vi "GamepadTeleop.vi"   [LabVIEW 2014]
uses:
  Elevator System/Typedef/TeirNumber.ctl
  <vilib>/Rock Robotics/WPI/Joystick/WPI_JoystickGetSetRefNum.vi
  Elevator System/Elevator System.lvlib
types:
  T1 = typedef "WPI_JoystickDevRef.ctl" = cluster{"Device":T2}
  T2 = typedef "WPI_JoystickDeviceEnum.ctl" = enum16{"USB 0", "USB 1", "USB 2", "USB 3", "USB 4", "USB 5"}
  T3 = typedef "Elevator System.lvlib/TeirNumber.ctl" = enum16{"T1", "T2", "T3", "T4", "T5", "T6"}
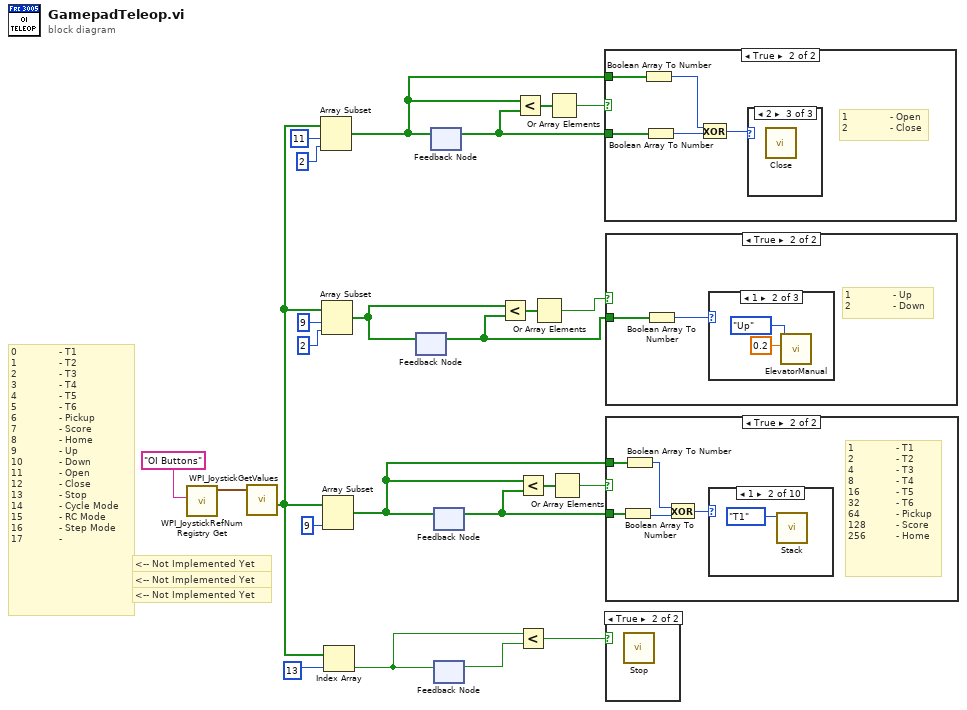
[diagram p0: block diagram]
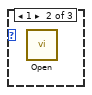
[diagram p4: hidden frame]
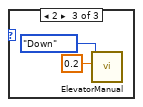
[diagram p8: hidden frame]
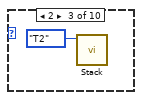
[diagram p11: hidden frame]
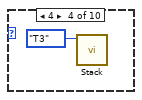
[diagram p12: hidden frame]
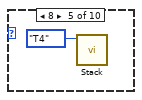
[diagram p13: hidden frame]
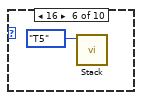
[diagram p14: hidden frame]
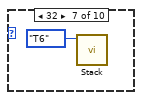
[diagram p15: hidden frame]
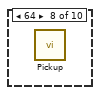
[diagram p16: hidden frame]
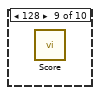
[diagram p17: hidden frame]
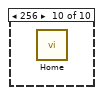
[diagram p18: hidden frame]
diagram:
  # "<-- Not Implemented Yet"
  # "<-- Not Implemented Yet"
  # "<-- Not Implemented Yet"
  # "0              - T1\n1              - T2\n2              - T3\n3              - T4\n4              - T5\n5              - T6\n6              - Pickup\n7              - Score\n8              - Home\n9              - Up\n10            - Down\n11            - Open\n12            - Close\n13            - Stop \n14            - Cycle Mode \n15            - RC Mode\n16            - Step Mode\n17            -"
  n1 = call <vilib>:"WPI_JoystickRefNum Registry Get.vi"("refnum name"="OI Buttons") -> ("JoystickDevRef"=w23:T1)  [unwired: 1 in, 9 out]
  n2 = call <vilib>:"WPI_JoystickGetValues.vi"("JoystickDevRef"=w23) -> ("Buttons"=w7:bool[])  [unwired: 6 in, 4 out]
  n3 = Array Subset(array=w7, index=11 ("length"), length=2) -> (w6:bool[])
  n4 = Array Subset(array=w7, index=9 ("length"), length=2) -> (w3:bool[])
  n5 = Array Subset(array=w7, length=9) -> (w5:bool[])  [unwired: 1 in]
  n6 = Index Array(array=w7, index=13) -> (element=w14:bool)
  n7 = feedback #1() -> (w1:bool[])  [unwired: 1 in]
  n8 = feedback-in #1(w3) -> ()
  n9 = feedback #2() -> (w9:bool[])  [unwired: 1 in]
  n10 = feedback-in #2(w6) -> ()
  n11 = feedback #3() -> (w20:bool[])  [unwired: 1 in]
  n12 = feedback-in #3(w5) -> ()
  n13 = feedback #4() -> (w15:bool)  [unwired: 1 in]
  n14 = feedback-in #4(w14) -> ()
  n15 = Less?(x=w3, y=w1) -> (x < y?=w4:bool[])
  n16 = Less?(x=w6, y=w9) -> (x < y?=w11:bool[])
  n17 = Less?(x=w5, y=w20) -> (x < y?=w22:bool[])
  n18 = Less?(x=w14, y=w15) -> (x < y?=w13:bool)
  n19 = Or Array Elements(Boolean array=w4) -> (logical OR=w2:bool)
  n20 = Or Array Elements(Boolean array=w11) -> (logical OR=w10:bool)
  n21 = Or Array Elements(Boolean array=w22) -> (logical OR=w21:bool)
  n22 = case shown="True" w10 {
    tunnel: w9 -> [_ w29]
    tunnel: w6 -> [_ w25]
    frame False {
    }
    frame True {
      # "1              - Open\n2              - Close"
      n23 = Boolean Array To Number(Boolean array=w25) -> (number=w26:u32)
      n24 = Boolean Array To Number(Boolean array=w29) -> (number=w27:u32)
      n25 = Exclusive Or(1:w27, 2:w26) -> (0:w28:u32)
      n26 = case shown="2" w28 {
        frame 0, Default {
        }
        frame 1 {
          n27 = call "Open.vi"() -> ()  [unwired: 12 in]
        }
        frame 2 {
          n28 = call "Close.vi"() -> ()  [unwired: 12 in]
        }
      }
    }
  }
  n29 = case shown="True" w2 {
    tunnel: w1 -> [_ w30]
    frame False {
    }
    frame True {
      # "1              - Up\n2              - Down"
      n30 = Boolean Array To Number(Boolean array=w30) -> (number=w31:u32)
      n31 = case shown="1" w31 {
        frame 0, Default {
        }
        frame 1 {
          n32 = call "ElevatorManual.vi"("Amount"=0.2, "Enum"=enum16{"Up", "Down"}."Up") -> ()  [unwired: 10 in]
        }
        frame 2 {
          n33 = call "ElevatorManual.vi"("Amount"=0.2, "Enum"=enum16{"Up", "Down"}."Down") -> ()  [unwired: 10 in]
        }
      }
    }
  }
  n34 = case shown="True" w21 {
    tunnel: w20 -> [_ w40]
    tunnel: w5 -> [_ w39]
    frame False {
    }
    frame True {
      # "1              - T1\n2              - T2\n4              - T3\n8              - T4\n16            - T5\n32            - T6\n64            - Pickup\n128          - Score\n256          - Home"
      n35 = Boolean Array To Number(Boolean array=w40) -> (number=w38:u32)
      n36 = Boolean Array To Number(Boolean array=w39) -> (number=w37:u32)
      n37 = Exclusive Or(1:w38, 2:w37) -> (0:w36:u32)
      n38 = case shown="1" w36 {
        frame 0, Default {
        }
        frame 1 {
          n39 = call "Stack.vi"("Teir"=TeirNumber."T1") -> ()  [unwired: 11 in]
        }
        frame 2 {
          n40 = call "Stack.vi"("Teir"=TeirNumber."T2") -> ()  [unwired: 11 in]
        }
        frame 4 {
          n41 = call "Stack.vi"("Teir"=TeirNumber."T3") -> ()  [unwired: 11 in]
        }
        frame 8 {
          n42 = call "Stack.vi"("Teir"=TeirNumber."T4") -> ()  [unwired: 11 in]
        }
        frame 16 {
          n43 = call "Stack.vi"("Teir"=TeirNumber."T5") -> ()  [unwired: 11 in]
        }
        frame 32 {
          n44 = call "Stack.vi"("Teir"=TeirNumber."T6") -> ()  [unwired: 11 in]
        }
        frame 64 {
          n45 = call "Pickup.vi"() -> ()  [unwired: 12 in]
        }
        frame 128 {
          n46 = call "Score.vi"() -> ()  [unwired: 12 in]
        }
        frame 256 {
          n47 = call "Home.vi"() -> ()  [unwired: 12 in]
        }
      }
    }
  }
  n48 = case shown="True" w13 {
    frame False {
    }
    frame True {
      n49 = call "Stop.vi"() -> ()  [unwired: 12 in]
    }
  }
